vi "Main.vi"() -> ()   [LabVIEW 2023]
uses:
  States.ctl
  System Data.ctl
  <vilib>/NI/Modbus Library/API/Master/Modbus Master.lvclass
  79a3c456-e4cd-4138-946e-1f307a576655.vi
  44454701-22d1-495e-97a7-b05a01e852b1.vi
  201a4777-ac33-490a-a616-c2a30b6a5525.vi
  0b243ea3-5714-4a42-89da-e34ccc22f44d.vi
  d4d9ab7c-afa5-4cc4-8e9e-5fa7235f49d3.vi
  d383db1f-ab98-46e8-8b04-d05cf59c4aeb.vi
  <vilib>/Utility/config.llb/Read Key (String).vi
  RS485/RS485.lvlib
  <vilib>/Utility/config.llb/NI_LVConfig.lvlib
  Arduino code/Serial_communication.lvlib
panel:
  in  "Izabrana varijanta":string
  in  "Select Variant":bool=TRUE
  in  "Status":bool
  in  "Stop":bool
  out "error out":errorcluster
  in  "Test":T1(array[cluster])
  in  "Dostupne varijante":string(combo)
  in  "error in":errorcluster
  in  "START":bool
  out "Monitor":string
  # "Ime testa"
  # "Donja \ngranica"
  # "Izmerena\nvrednost"
  # "Gornja \ngranica"
  # "Rezultat\ntesta"
  # "Rezultat testiranja :"
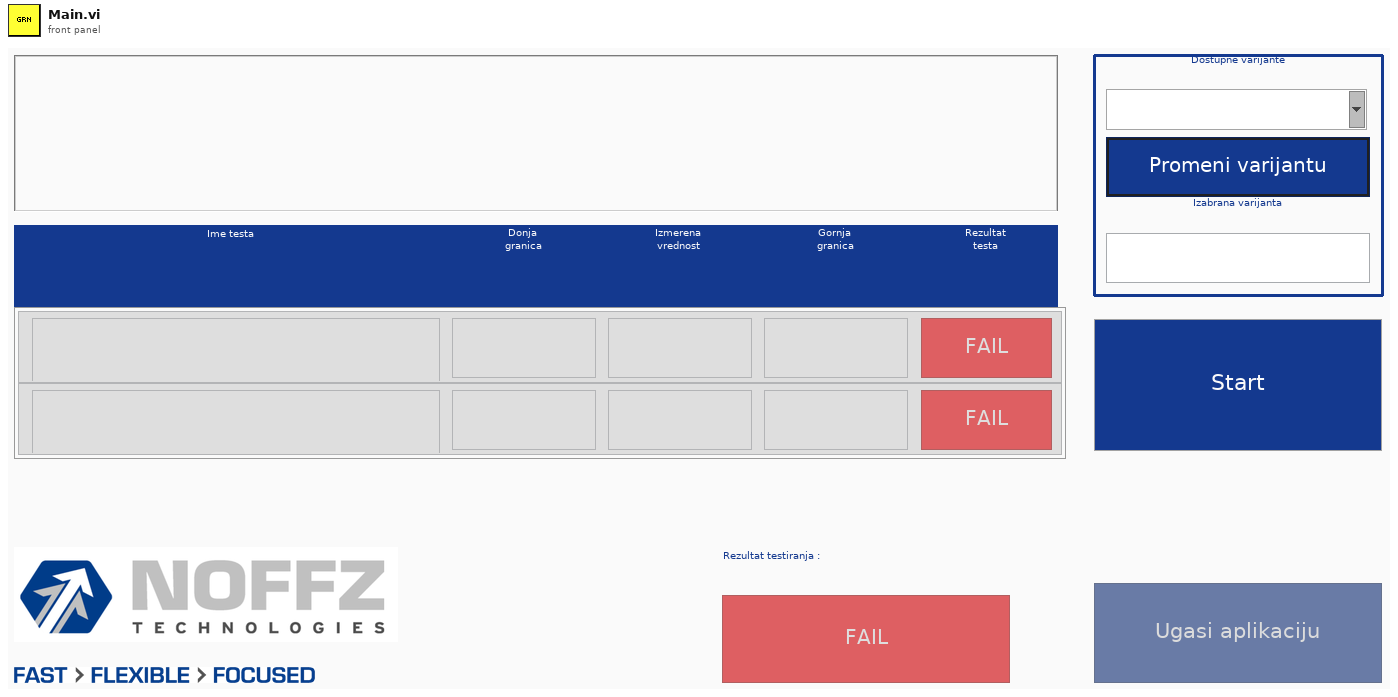
[diagram p1: front panel]
types:
  T1 = cluster{"TestName":string, "LOW":string, "MEAS":string, "HIGH":string, "Status":bool}[]
  T2 = cluster{"TestName":string, "LOW":string, "MEAS":string, "HIGH":string, "STATUS":bool}[]
  T3 = typedef "System Data.ctl" = cluster{"RS485 reference":refnum<class "Modbus Master.lvclass">, "Testing Status":bool, "Selected Variant":string, "Number Of tests":i32, "Test Names":string[], "Test Results":bool[], "Test Limits":cluster{"Low Limit":dbl, "High Limit":dbl, "GELE":bool}[], "Current test":i32, "Test Values":dbl[], "ArduinoRef":refnum<visa-resource-name>}
  T4 = typedef "States.ctl" = enum16{"Initialize", "Select Variant", "Idle", "Start Test", "Test", "Result", "Deinitialize"}
  T5 = enum8{"Enabled", "Disabled", "Disabled and Grayed Out"}
  T6 = cluster{"TestName":string, "LOW":string, "MEAS":string, "HIGH":string, "Status":bool}
  T7 = cluster{"TestName":string, "LOW":string, "MEAS":string, "HIGH":string, "STATUS":bool}
  T8 = typedef "NI_LVConfig.lvlib/Config Data RefNum.ctl" = refnum<k1>
  T9 = cluster{"Low Limit":dbl, "High Limit":dbl, "GELE":bool}[]
  T10 = cluster{"Low Limit":dbl, "High Limit":dbl, "GELE":bool}
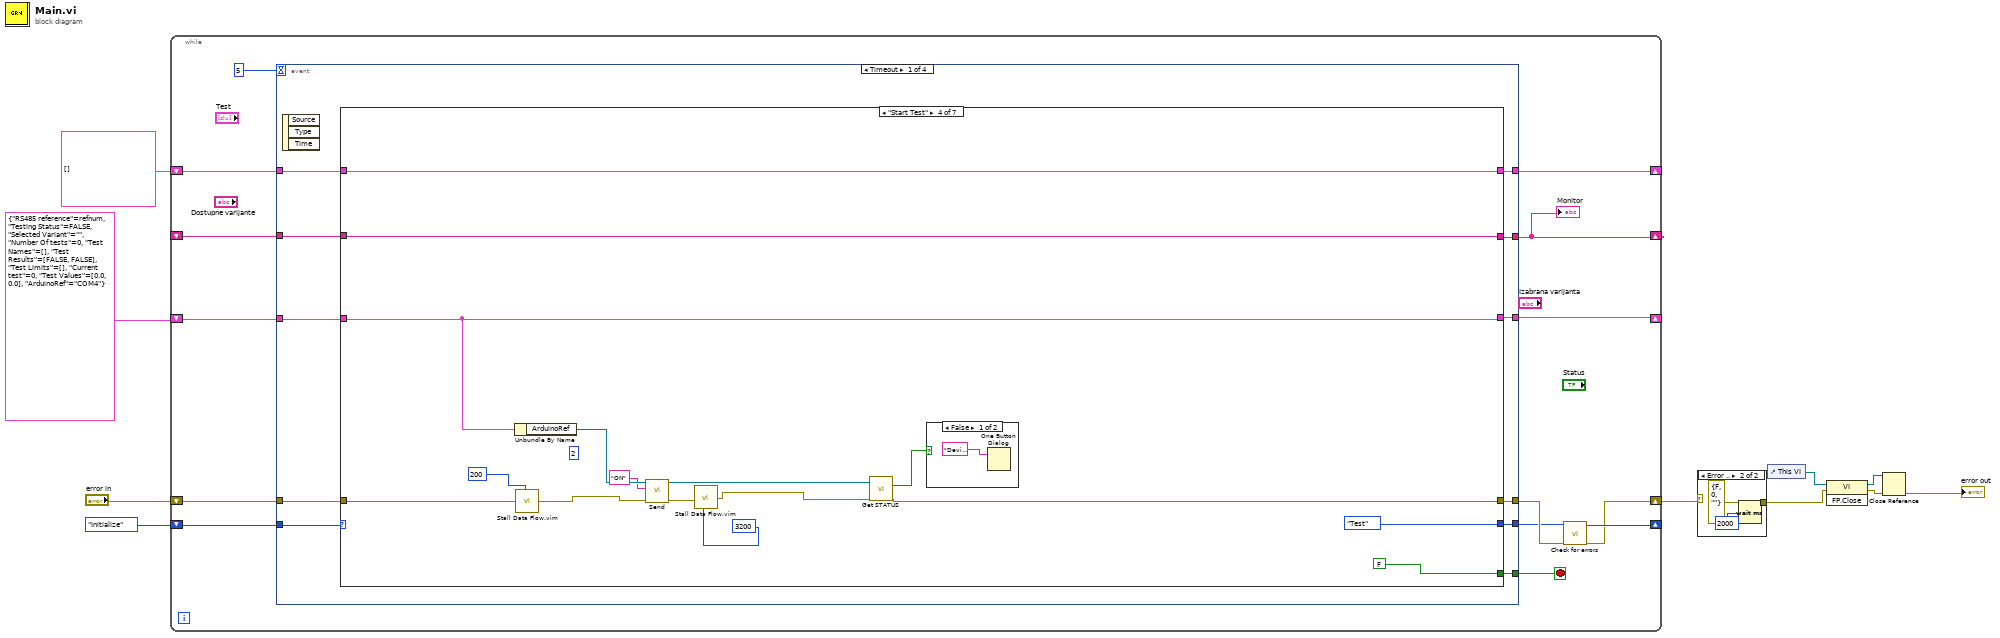
[diagram p0: block diagram]
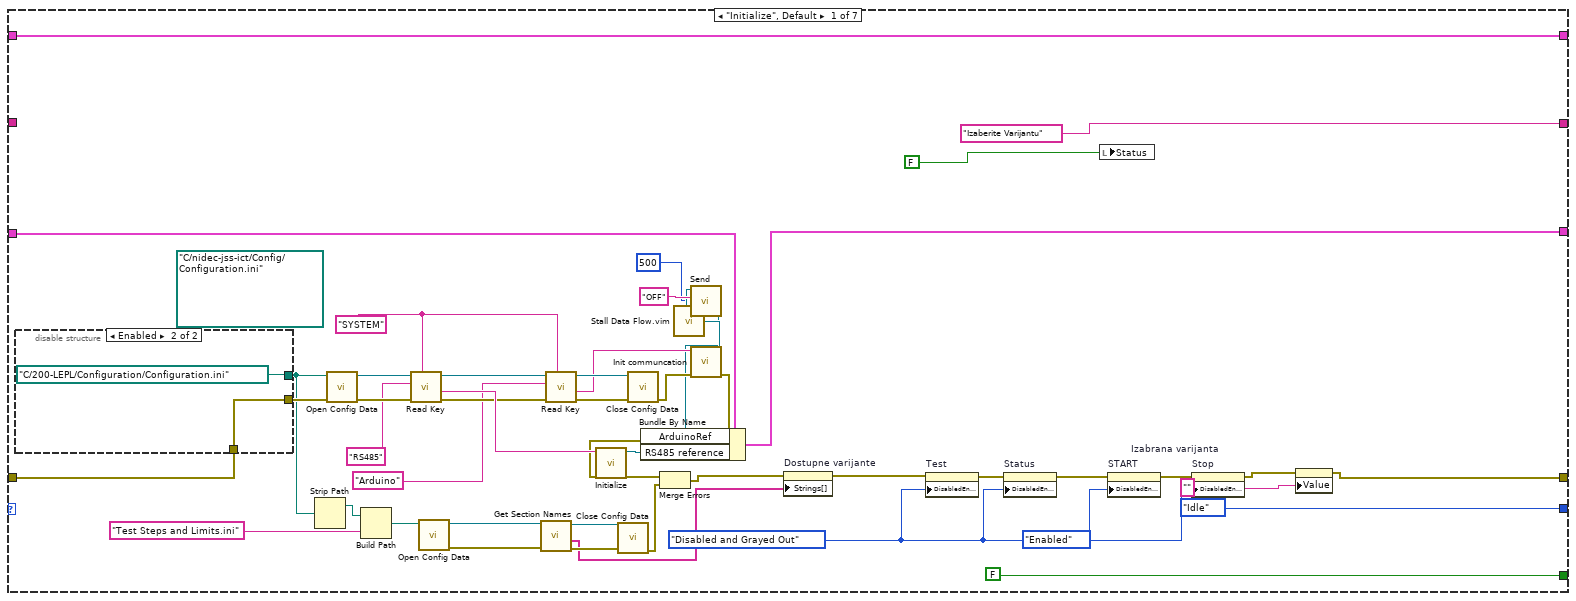
[diagram p3: hidden frame]
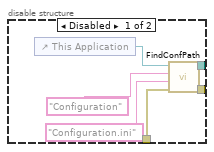
[diagram p4: hidden frame]
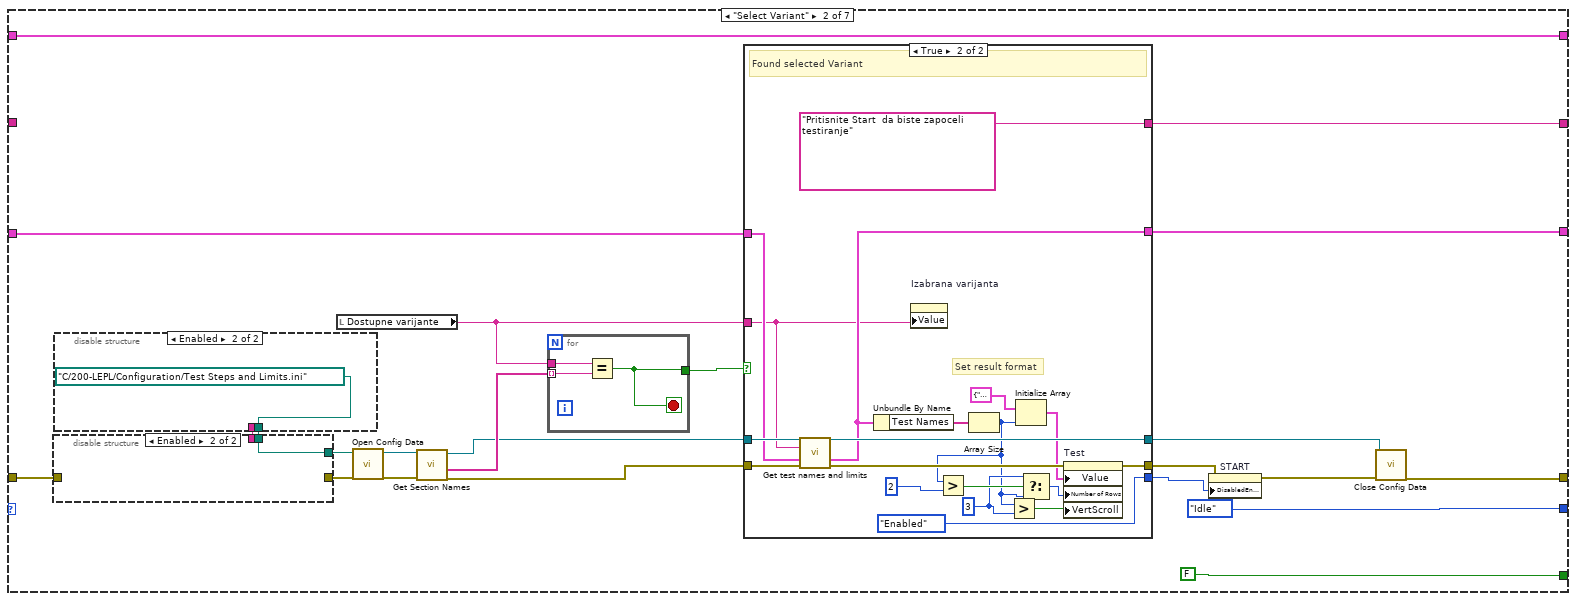
[diagram p5: hidden frame]
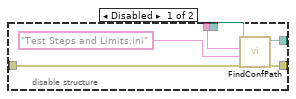
[diagram p6: hidden frame]
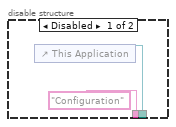
[diagram p7: hidden frame]
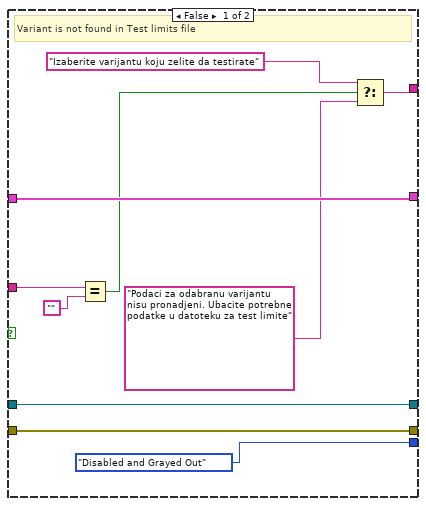
[diagram p8: hidden frame]
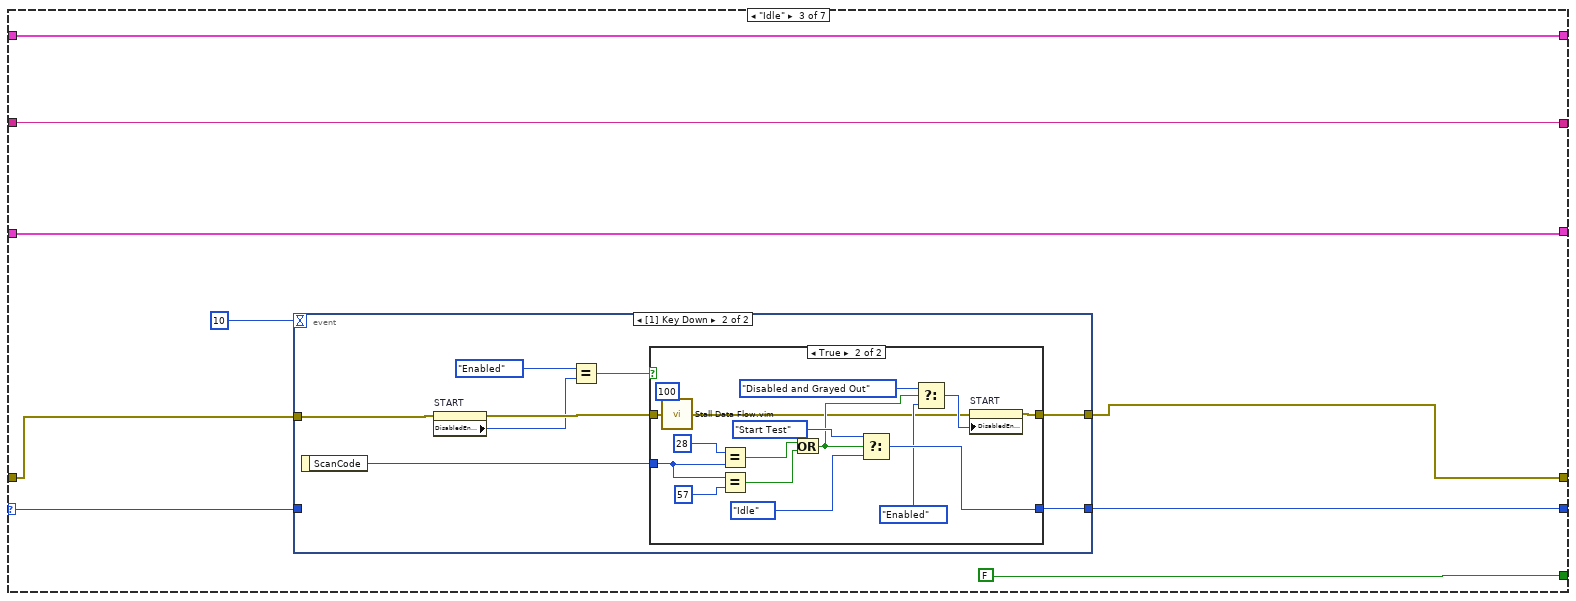
[diagram p9: hidden frame]
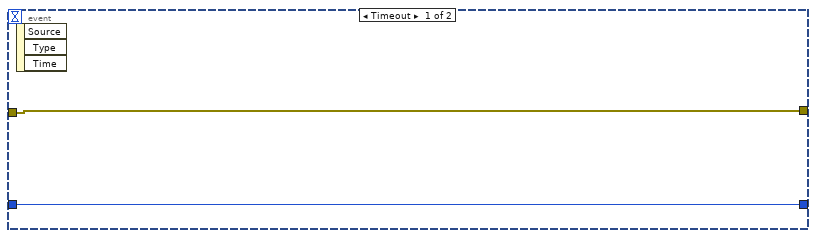
[diagram p10: hidden frame]
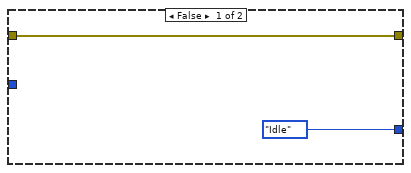
[diagram p11: hidden frame]
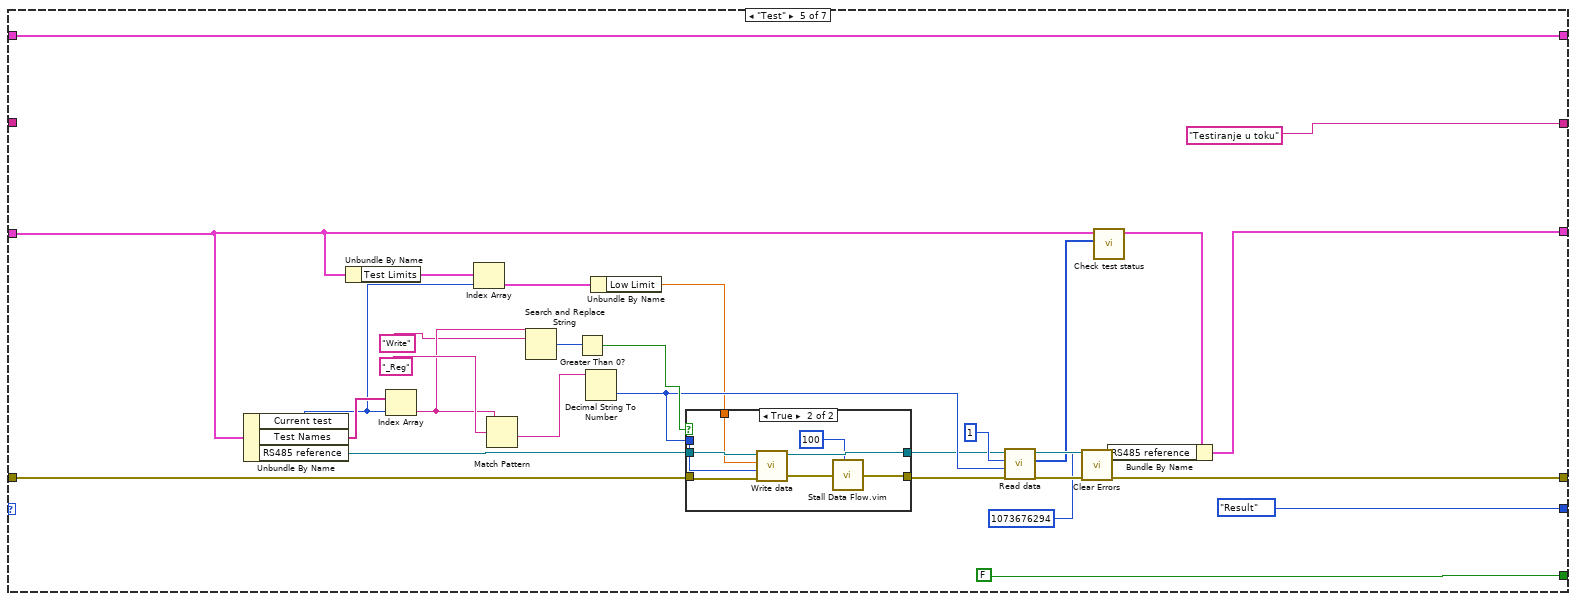
[diagram p13: hidden frame]
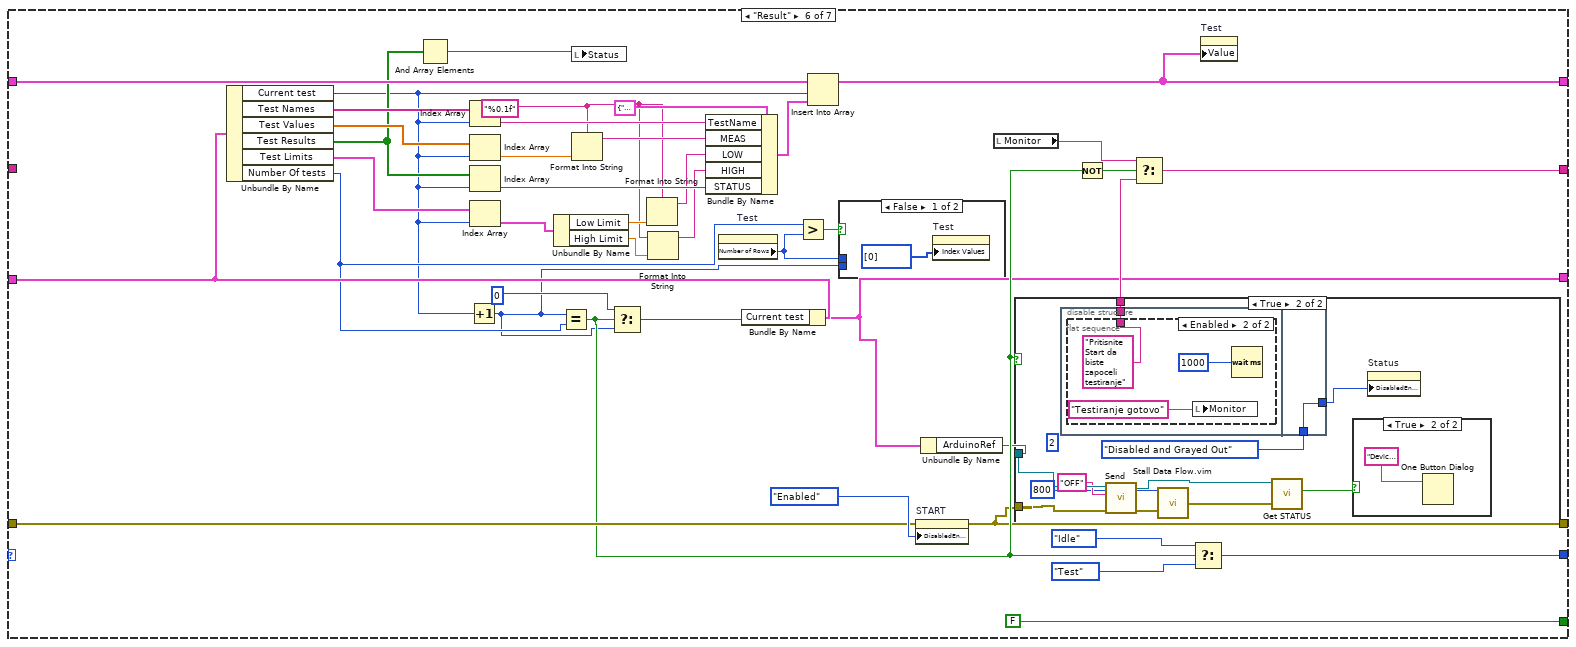
[diagram p15: hidden frame]
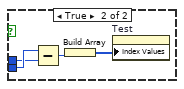
[diagram p16: hidden frame]
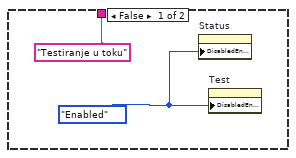
[diagram p17: hidden frame]
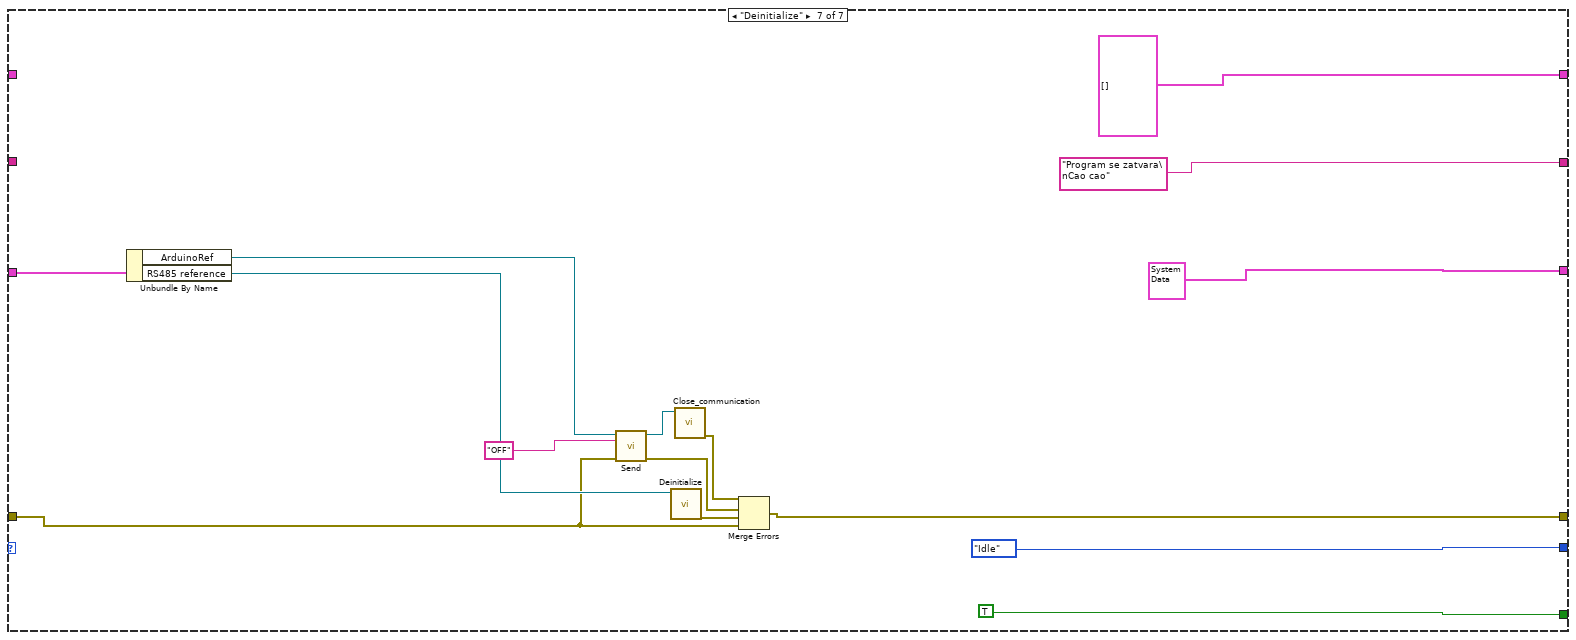
[diagram p20: hidden frame]
diagram:
  n1 = while {
    shift-right: [w12] -> w3
    shift-left: "error in" -> [w22]
    shift-right: [w20] -> _
    shift-left: T3 {"RS485 reference"=refnum, "Testing Status"=FALSE, "Selected Variant"="", "Number Of tests"=0, "Test Names"=[], "Test Results"=[FALSE, FALSE], "Test Limits"=[], "Current test"=0, "Test Values"=[0.0, 0.0], "ArduinoRef"="COM4"} -> [w21]
    shift-right: [w16] -> _
    shift-left: States."Initialize" -> [w23]
    shift-right: [w11] -> _
    shift-left: T2 [] ("Test") -> [w15]
    shift-right: [w14] -> _
    shift-left: _ -> [w13]
    stop <- w19 stop-if-true
    n2 = event shown="[0] Timeout" {
      selector: _ -> [_ _ _ _]
      dyn-events: _ -> [_ _ _ _]
      timeout: 5 -> [_ _ _ _]
      tunnel: w23 -> [w35 _ _ _]
      tunnel: w22 -> [w34 w334 w341 w347]
      tunnel: w21 -> [w33 w333 w342 w350]
      tunnel: [w32 w334 w340 w346] -> w18
      tunnel: [w31 w333 w342 w350] -> w20
      tunnel: [w30 FALSE FALSE FALSE] -> w19
      tunnel: [w29 States."Select Variant" States."Start Test" States."Deinitialize"] -> w17
      tunnel: [w28 w331 w338 w349] -> w11
      tunnel: w15 -> [w27 w331 w338 w349]
      tunnel: [w26 w332 w337 w348] -> w14
      tunnel: w13 -> [w25 w332 w337 w348]
      event Timeout {
        n3 = event-data() -> ()  [unwired: 1 in, 3 out]
        n4 = case shown="\"Start Test\"" w35 {
          selector: w35 -> [_ _ w158 _ _ _ _]
          tunnel: w34 -> [w72 w113 w161 w201 w217 w289 w318]
          tunnel: w33 -> [w79 w105 w166 w208 w222 w273 w327]
          tunnel: [w50 w103 w160 w203 w213 w253 w323] -> w32
          tunnel: [w77 w104 w166 w208 w233 w252 T3 {"RS485 reference"=refnum, "Testing Status"=FALSE, "Selected Variant"="", "Number Of tests"=0, "Test Names"=[], "Test Results"=[], "Test Limits"=[], "Current test"=0, "Test Values"=[], "ArduinoRef"="COM4"}] -> w31
          tunnel: [FALSE FALSE FALSE FALSE FALSE FALSE TRUE] -> w30
          tunnel: [States."Idle" States."Idle" w159 States."Test" States."Result" w268 States."Idle"] -> w29
          tunnel: [w58 w94 w164 w210 w238 w259 T2 [] ("Test")] -> w28
          tunnel: w27 -> [w58 w94 w164 w210 w238 w288 _]
          tunnel: ["Izaberite Varijantu" ("Monitor") w93 w163 w209 "Testiranje u toku" ("message") w266 "Program se zatvara\nCao cao" ("message")] -> w26
          tunnel: w25 -> [_ _ w163 w209 _ _ _]
          frame "Initialize", Default {
            w53 = T5."Disabled and Grayed Out" ("Disabled")
            w44 = "SYSTEM" ("key")
            (unwired) path "C:/nidec-jss-ict/Config/Configuration.ini" ("configuration file path")
            n5 = disable-structure shown="Enabled" {
              disable-tunnel: [w88 w92] -> w84
              disable-tunnel: w72 -> [w87 w92]
              disable-tunnel: [w85 path "C:/200-LEPL/Configuration/Configuration.ini" ("conf path")] -> w71
              frame Disabled {
                n6 = control-ref of="This Application"() -> (w86:refnum<vi>)
                n7 = call "FindConfPath.vi"("error in"=w87, "FileName"="Configuration.ini", "SubFolder"="Configuration", "Application in"=w86) -> ("error out"=w88:errorcluster, "conf path"=w85:path)  [unwired: 6 in]
              }
              frame Enabled {
              }
            }
            n8 = Strip Path(path=w71) -> (stripped path=w70:path)  [unwired: 1 out]
            n9 = call <vilib>:"Open Config Data.vi"("error in (no error)"=w84, "configuration file path"=w71) -> ("error out"=w82:errorcluster, "refnum"=w83:T8)  [unwired: 7 in, 1 out]
            n10 = Build Path(base path=w70, name or relative path="Test Steps and Limits.ini" ("FileName")) -> (appended path=w68:path)
            n11 = call-poly <vilib>:"Read Key.vi"("section"=w44, "error in (no error)"=w82, "key"="RS485" ("default value"), "refnum"=w83) -> ("error out"=w47:errorcluster, "value"=w80:string, "refnum out"=w49:T8)  [unwired: 4 in, 1 out]
            n12 = call <vilib>:"Open Config Data.vi"("configuration file path"=w68) -> ("error out"=w74:errorcluster, "refnum"=w73:T8)  [unwired: 8 in, 1 out]
            n13 = call <vilib>:"Get Section Names.vi"("error in (no error)"=w74, "refnum"=w73) -> ("error out"=w67:errorcluster, "section names"=w63:string[], "refnum out"=w66:T8)  [unwired: 7 in]
            n14 = call-poly <vilib>:"Read Key.vi"("section"=w44, "error in (no error)"=w47, "key"="Arduino", "refnum"=w49) -> ("error out"=w46:errorcluster, "value"=w41:string, "refnum out"=w48:T8)  [unwired: 4 in, 1 out]
            n15 = call <vilib>:"Close Config Data.vi"("error in (no error)"=w67, "refnum"=w66) -> ("error out"=w64:errorcluster)  [unwired: 8 in, 1 out]
            n16 = call <vilib>:"Close Config Data.vi"("error in (no error)"=w46, "refnum"=w48) -> ("error out"=w43:errorcluster)  [unwired: 8 in, 1 out]
            n17 = call "Init communcation.vi"("error in (no error)"=w43, "COM port"=w41) -> ("error out"=w42:errorcluster, "VISA Refnum out"=w40:refnum<visa-resource-name>)  [unwired: 8 in]
            n18 = call "Initialize.vi"("error in"=w42, "NI name"=w80) -> ("error out"=w65:errorcluster, "Modbus master out"=w78:refnum<class "Modbus Master.lvclass">)  [unwired: 8 in]
            n19 = Merge Errors(w65, w64) -> (w57:errorcluster)
            n20 = call "Stall Data Flow.vim"("value in"=w40, "milliseconds to wait"=u32 500) -> ("value out"=w37:refnum<visa-resource-name>)  [unwired: 1 out]
            n21 = call "Send.vi"("Command"="OFF", "VISA Refnum in"=w37) -> ("VISA Refnum out"=w39:refnum<visa-resource-name>)  [unwired: 8 in, 1 out]
            n22 = Bundle By Name(cluster=w79, "ArduinoRef"=w39, "RS485 reference"=w78) -> (w77:T3)
            n23 = property on="Dostupne varijante" class="CmbBox"(error in=w57, "Strings[]"=w63) -> (error out=w55:errorcluster)  [unwired: 1 in, 1 out]
            n24 = property on="Test" class="Arr (strict)"(error in=w55, "DisabledEnum"=w53) -> (error out=w56:errorcluster)  [unwired: 1 in, 1 out]
            n25 = property on="Status" class="Bool (strict)"(error in=w56, "DisabledEnum"=w53) -> (error out=w54:errorcluster)  [unwired: 1 in, 1 out]
            n26 = local write "Status"(FALSE ("REZULTAT TESTIRANJA :")) -> ()
            n27 = property on="START" class="Bool"(error in=w54, "DisabledEnum"=w53) -> (error out=w60:errorcluster)  [unwired: 1 in, 1 out]
            n28 = property on="Stop" class="Bool"(error in=w60, "DisabledEnum"=T5."Enabled" ("Disabled")) -> (error out=w51:errorcluster)  [unwired: 1 in, 1 out]
            n29 = property on="Izabrana varijanta" class="Str"(error in=w51, "Value"="" ("Izabrana varijanta")) -> (error out=w50:errorcluster)  [unwired: 1 in, 1 out]
          }
          frame "Select Variant" {
            n30 = disable-structure shown="Enabled" {
              disable-tunnel: ["Configuration" ("SubFolder") _] -> w115
              disable-tunnel: [w123 path "C:/200-LEPL/Configuration/Test Steps and Limits.ini" ("conf path")] -> w114
              frame Disabled {
                n31 = control-ref of="This Application"() -> (w123:refnum<vi>)
              }
              frame Enabled {
              }
            }
            n32 = disable-structure shown="Enabled" {
              disable-tunnel: w115 -> [w121 _]
              disable-tunnel: w114 -> [w119 w122]
              disable-tunnel: w113 -> [w118 _]
              disable-tunnel: [w117 w122] -> w112
              disable-tunnel: [w116 _] -> w111
              frame Disabled {
                n33 = call "FindConfPath.vi"("error in"=w118, "FileName"="Test Steps and Limits.ini", "SubFolder"=w121, "Application in"=w119) -> ("error out"=w116:errorcluster, "conf path"=w117:path)  [unwired: 6 in]
              }
              frame Enabled {
              }
            }
            n34 = local read "Dostupne varijante"() -> (w106:string)
            n35 = call <vilib>:"Open Config Data.vi"("error in (no error)"=w111, "configuration file path"=w112) -> ("error out"=w110:errorcluster, "refnum"=w109:T8)  [unwired: 7 in, 1 out]
            n36 = call <vilib>:"Get Section Names.vi"("error in (no error)"=w110, "refnum"=w109) -> ("error out"=w95:errorcluster, "section names"=w108:string[], "refnum out"=w107:T8)  [unwired: 7 in]
            n37 = for {
              tunnel: w108 -> [w157] mode=indexing
              tunnel: w106 -> [w156]
              tunnel: [w155] -> w99
              stop <- w155 stop-if-true
              n38 = Equal?(x=w156, y=w157) -> (x = y?=w155:bool)
            }
            n39 = case shown="True" w99 {
              tunnel: w107 -> [w135 w154]
              tunnel: w106 -> [w131 w136]
              tunnel: w105 -> [w134 w150]
              tunnel: [w134 w148] -> w104
              tunnel: [w132 w146] -> w98
              tunnel: [w135 w153] -> w102
              tunnel: [T5."Disabled and Grayed Out" ("Disabled") T5."Enabled" ("Disabled")] -> w96
              tunnel: w95 -> [w132 w151]
              tunnel: [w127 "Pritisnite Start  da biste zapoceli testiranje" ("message")] -> w93
              frame False {
                # "Variant is not found in Test limits file"
                n40 = Equal?(x=w131, y="") -> (x = y?=w129:bool)
                n41 = Select(t="Izaberite varijantu koju zelite da testirate", s=w129, f="Podaci za odabranu varijantu nisu pronadjeni. Ubacite potrebne podatke u datoteku za test limite" ("message")) -> (s? t:f=w127:string)
              }
              frame True {
                w139 = 3 ("y")
                # "Set result format"
                # "Found selected Variant"
                n42 = call "Get test names and limits.vi"("Refnum in"=w154, "Variant"=w136, "System data in"=w150, "error in"=w151) -> ("Refnum out"=w153:T8, "System data out"=w148:T3, "error out"=w147:errorcluster)  [unwired: 9 in]
                n43 = Unbundle By Name(w148) -> ("Test Names"=w145:string[])
                n44 = property on="Izabrana varijanta" class="Str"("Value"=w136) -> ()  [unwired: 2 in, 2 out]
                n45 = Array Size(array=w145) -> (size(s)=w138:i32)
                n46 = Greater?(x=w138, y=2) -> (0:w140:bool)
                n47 = Greater?(x=w138, y=w139) -> (0:w142:bool)
                n48 = Initialize Array(T6 {"TestName"="", "LOW"="", "MEAS"="", "HIGH"="", "Status"=FALSE} ("Test"), w138) -> (w143:T1)
                n49 = Select(t=w139, s=w140, f=w138) -> (s? t:f=w137:i32)
                n50 = property on="Test" class="Arr (strict)"(error in=w147, "Value"=w143, "Number of Rows"=w137, "VertScroll"=w142) -> (error out=w146:errorcluster)  [unwired: 1 in, 1 out]
              }
            }
            n51 = property on="START" class="Bool"(error in=w98, "DisabledEnum"=w96) -> (error out=w97:errorcluster)  [unwired: 1 in, 1 out]
            n52 = call <vilib>:"Close Config Data.vi"("error in (no error)"=w97, "refnum"=w102) -> ("error out"=w103:errorcluster)  [unwired: 8 in, 1 out]
          }
          frame "Idle" {
            n53 = event shown="[1] Key Down" {
              selector: _ -> [_ _]
              dyn-events: _ -> [_ _]
              timeout: 10 -> [_ _]
              tunnel: w161 -> [w167 w169]
              tunnel: [w167 w173] -> w160
              tunnel: [w168 w172] -> w159
              tunnel: w158 -> [w168 _]
              event Timeout {
                n54 = event-data() -> ()  [unwired: 1 in, 3 out]
              }
              event Key Down {
                n55 = event-data() -> ("ScanCode"=w174:i16)  [unwired: 1 in]
                n56 = property on="START" class="Bool"(error in=w169) -> (error out=w171:errorcluster, "DisabledEnum"=w170:T5)  [unwired: 1 in, 1 out]
                n57 = Equal?(x=T5."Enabled", y=w170) -> (x = y?=w175:bool)
                n58 = case shown="True" w175 {
                  tunnel: w174 -> [_ w189]
                  tunnel: [States."Idle" w190] -> w172
                  tunnel: w171 -> [w177 w186]
                  tunnel: [w177 w185] -> w173
                  frame False {
                  }
                  frame True {
                    n59 = call "Stall Data Flow.vim"("value in"=w186, "milliseconds to wait"=u32 100) -> ("value out"=w180:errorcluster)  [unwired: 1 out]
                    n60 = Equal?(x=i16 28, y=w189) -> (x = y?=w192:bool)
                    n61 = Equal?(x=w189, y=i16 57 ("x")) -> (x = y?=w191:bool)
                    n62 = Or(x=w192, y=w191) -> (x .or. y?=w183:bool)
                    n63 = Select(t=States."Start Test", s=w183, f=States."Idle") -> (s? t:f=w190:T4)
                    n64 = Select(t=T5."Disabled and Grayed Out" ("Disabled"), s=w183, f=T5."Enabled" ("Disabled")) -> (s? t:f=w181:T5)
                    n65 = property on="START" class="Bool"(error in=w180, "DisabledEnum"=w181) -> (error out=w185:errorcluster)  [unwired: 1 in, 1 out]
                  }
                }
              }
            }
          }
          frame "Start Test" {
            (unwired) 2
            n66 = Unbundle By Name(w208) -> ("ArduinoRef"=w205:refnum<visa-resource-name>)
            n67 = call "Stall Data Flow.vim"("value in"=w201, "milliseconds to wait"=u32 200) -> ("value out"=w197:errorcluster)  [unwired: 1 out]
            n68 = call "Send.vi"("error in (no error)"=w197, "Command"="ON", "VISA Refnum in"=w205) -> ("error out"=w195:errorcluster, "VISA Refnum out"=w204:refnum<visa-resource-name>)  [unwired: 7 in]
            n69 = call "Stall Data Flow.vim"("value in"=w195, "milliseconds to wait"=u32 3200) -> ("value out"=w198:errorcluster)  [unwired: 1 out]
            n70 = call "Get STATUS.vi"("error in (no error)"=w198, "VISA Refnum in"=w204) -> ("error out"=w203:errorcluster, "LED ON"=w202:bool)  [unwired: 6 in, 2 out]
            n71 = case shown="False" w202 {
              frame False {
                n72 = One Button Dialog(message="Device did not turn ON. Please close the program and open it again") -> ()  [unwired: 1 in, 1 out]
              }
              frame True {
              }
            }
          }
          frame "Test" {
            n73 = Unbundle By Name(w222) -> ("Current test"=w220:i32, "Test Names"=w237:string[], "RS485 reference"=w224:refnum<class "Modbus Master.lvclass">)
            n74 = Unbundle By Name(w222) -> ("Test Limits"=w221:T9)
            n75 = Index Array(array=w237, index=w220) -> (element=w228:string)
            n76 = Index Array(array=w221, index=w220) -> (element=w219:T10)
            n77 = Match Pattern(string=w228, regular expression="_Reg") -> (after substring=w235:string)  [unwired: 1 in, 3 out]
            n78 = Search and Replace String(input string=w228, search string="Write") -> (number of replacements=w226:i32)  [unwired: 6 in, 3 out]
            n79 = Greater Than 0?(x=w226) -> (x > 0?=w225:bool)
            n80 = Decimal String To Number(string=w235) -> (number=w223:i32)  [unwired: 2 in, 1 out]
            n81 = Unbundle By Name(w219) -> ("Low Limit"=w218:dbl)
            n82 = case shown="True" w225 {
              tunnel: w224 -> [w242 w250]
              tunnel: [w242 w249] -> w215
              tunnel: w223 -> [_ w248]
              tunnel: w218 -> [_ w247]
              tunnel: w217 -> [w241 w246]
              tunnel: [w241 w244] -> w214
              frame False {
              }
              frame True {
                n83 = call "Write data.vi"("error in"=w246, "starting address"=w248, "register value to write"=w247, "Modbus master in"=w250) -> ("error out"=w245:errorcluster, "Modbus master out"=w249:refnum<class "Modbus Master.lvclass">)  [unwired: 6 in]
                n84 = call "Stall Data Flow.vim"("value in"=w245, "milliseconds to wait"=u32 100) -> ("value out"=w244:errorcluster)  [unwired: 1 out]
              }
            }
            n85 = call "Read data.vi"("error in"=w214, "starting address"=w223, "number of inputs"=u16 1, "Modbus master in"=w215) -> ("error out"=w234:errorcluster, "register values"=w230:u16[], "Modbus master out"=w232:refnum<class "Modbus Master.lvclass">)  [unwired: 5 in]
            n86 = call <vilib>:"Clear Errors.vi"("error in (no error)"=w234, "specific error code to clear (0: all)"=1073676294) -> ("error out"=w213:errorcluster)  [unwired: 4 in, 1 out]
            n87 = call "Check test status.vi"("register values"=w230, "System data in"=w222) -> ("System data out"=w231:T3)  [unwired: 9 in]
            n88 = Bundle By Name(cluster=w231, "RS485 reference"=w232) -> (w233:T3)
          }
          frame "Result" {
            w263 = "%0.1f" ("format string")
            n89 = Unbundle By Name(w273) -> ("Current test"=w256:i32, "Test Names"=w286:string[], "Test Values"=w284:dbl[], "Test Results"=w264:bool[], "Test Limits"=w280:T9, "Number Of tests"=w258:i32)
            n90 = And Array Elements(Boolean array=w264) -> (logical AND=w265:bool)
            n91 = Increment(x=w256) -> (x+1=w255:i32)
            n92 = Index Array(array=w286, index=w256) -> (element=w285:string)
            n93 = Index Array(array=w284, index=w256) -> (element=w283:dbl)
            n94 = Index Array(array=w264, index=w256) -> (element=w281:bool)
            n95 = Index Array(array=w280, index=w256) -> (element=w279:T10)
            n96 = Unbundle By Name(w279) -> ("Low Limit"=w278:dbl, "High Limit"=w277:dbl)
            n97 = Equal?(x=w255, y=w258) -> (x = y?=w261:bool)
            n98 = local write "Status"(w265) -> ()
            n99 = Format Into String(format string=w263, w283) -> (resulting string=w282:string)  [unwired: 2 in, 1 out]
            n100 = Select(t=0, s=w261, f=w255) -> (s? t:f=w271:i32)
            n101 = Format Into String(format string=w263, w278) -> (resulting string=w276:string)  [unwired: 2 in, 1 out]
            n102 = Format Into String(format string=w263, w277) -> (resulting string=w275:string)  [unwired: 2 in, 1 out]
            n103 = Bundle By Name(cluster=T7 {"TestName"="", "LOW"="", "MEAS"="", "HIGH"="", "STATUS"=FALSE} ("new element/subarray"), "TestName"=w285, "MEAS"=w282, "LOW"=w276, "HIGH"=w275, "STATUS"=w281) -> (w274:T7)
            n104 = property on="Test" class="Arr (strict)"() -> ("Number of Rows"=w254:u32)  [unwired: 2 in, 2 out]
            n105 = Bundle By Name(cluster=w273, "Current test"=w271) -> (w252:T3)
            n106 = Greater?(x=w258, y=w254) -> (0:w257:bool)
            n107 = Insert Into Array(array=w288, index=w256, new element=w274) -> (w259:T2)
            n108 = case shown="False" w257 {
              tunnel: w255 -> [_ w296]
              tunnel: w254 -> [_ w295]
              frame False {
                n109 = property on="Test" class="Arr (strict)"("Index Values"=u32[] [0]) -> ()  [unwired: 2 in, 2 out]
              }
              frame True {
                n110 = Subtract(x=w296, y=w295) -> (x-y=w294:u32)
                n111 = Build Array(w294) -> (w293:u32[])
                n112 = property on="Test" class="Arr (strict)"("Index Values"=w293) -> ()  [unwired: 2 in, 2 out]
              }
            }
            n113 = property on="START" class="Bool"(error in=w289, "DisabledEnum"=T5."Enabled" ("Disabled")) -> (error out=w253:errorcluster)  [unwired: 1 in, 1 out]
            n114 = Unbundle By Name(w252) -> ("ArduinoRef"=w251:refnum<visa-resource-name>)
            n115 = local read "Monitor"() -> (w267:string)
            n116 = case shown="True" w261 {
              tunnel: ["Testiranje u toku" ("message") w309] -> w260
              tunnel: w253 -> [_ w302]
              tunnel: w251 -> [_ w306]
              frame False {
                w298 = T5."Enabled" ("Disabled")
                n117 = property on="Status" class="Bool (strict)"("DisabledEnum"=w298) -> ()  [unwired: 2 in, 2 out]
                n118 = property on="Test" class="Arr (strict)"("DisabledEnum"=w298) -> ()  [unwired: 2 in, 2 out]
              }
              frame True {
                (unwired) 2
                n119 = flat-sequence {
                  tunnel: [w311] -> w309
                  tunnel: [w315] -> w307
                  tunnel: T5."Disabled and Grayed Out" ("Disabled") -> [w315]
                  frame #0 {
                    n120 = disable-structure shown="Enabled" {
                      disable-tunnel: [_ "Pritisnite Start da biste zapoceli testiranje" ("message")] -> w311
                      frame Disabled {
                      }
                      frame Enabled {
                        n121 = local write "Monitor"("Testiranje gotovo" ("Monitor")) -> ()
                        n122 = Wait (ms)(milliseconds to wait=u32 1000) -> ()  [unwired: 1 out]
                      }
                    }
                  }
                  frame #1 {
                  }
                }
                n123 = call "Send.vi"("error in (no error)"=w302, "Command"="OFF", "VISA Refnum in"=w306) -> ("error out"=w300:errorcluster, "VISA Refnum out"=w305:refnum<visa-resource-name>)  [unwired: 7 in]
                n124 = call "Stall Data Flow.vim"("value in"=w300, "milliseconds to wait"=u32 800) -> ("value out"=w303:errorcluster)  [unwired: 1 out]
                n125 = call "Get STATUS.vi"("error in (no error)"=w303, "VISA Refnum in"=w305) -> ("LED ON"=w304:bool)  [unwired: 6 in, 3 out]
                n126 = case shown="True" w304 {
                  frame False {
                  }
                  frame True {
                    n127 = One Button Dialog(message="Device did not reset\nPlease close the prorgam and open it again") -> ()  [unwired: 1 in, 1 out]
                  }
                }
                n128 = property on="Status" class="Bool (strict)"("DisabledEnum"=w307) -> ()  [unwired: 2 in, 2 out]
              }
            }
            n129 = Not(x=w261) -> (.not. x?=w262:bool)
            n130 = Select(t=w267, s=w262, f=w260) -> (s? t:f=w266:string)
            n131 = Select(t=States."Idle", s=w261, f=States."Test") -> (s? t:f=w268:T4)
            n132 = property on="Test" class="Arr (strict)"("Value"=w259) -> ()  [unwired: 2 in, 2 out]
          }
          frame "Deinitialize" {
            n133 = Unbundle By Name(w327) -> ("ArduinoRef"=w321:refnum<visa-resource-name>, "RS485 reference"=w330:refnum<class "Modbus Master.lvclass">)
            n134 = call "Send.vi"("error in (no error)"=w318, "Command"="OFF", "VISA Refnum in"=w321) -> ("error out"=w316:errorcluster, "VISA Refnum out"=w320:refnum<visa-resource-name>)  [unwired: 7 in]
            n135 = call "Deinitialize.vi"("Modbus master in"=w330) -> ("error out"=w324:errorcluster)  [unwired: 10 in]
            n136 = call "Close_communication.vi"("VISA Refnum in"=w320) -> ("error out"=w317:errorcluster)  [unwired: 10 in]
            n137 = Merge Errors(w317, w316, w324, w318) -> (w323:errorcluster)
          }
        }
      }
      event "Select Variant": Value Change {
        n138 = event-data() -> ()  [unwired: 1 in, 6 out]
      }
      event "START": Value Change {
        n139 = event-data() -> ()  [unwired: 1 in, 2 out]
        n140 = property on="START" class="Bool"(error in=w341, "DisabledEnum"=T5."Disabled and Grayed Out" ("Disabled")) -> (error out=w340:errorcluster)  [unwired: 1 in, 1 out]
      }
      event "Stop": Value Change {
        n141 = event-data() -> ()  [unwired: 1 in, 6 out]
        n142 = property on="Stop" class="Bool"(error in=w347, "DisabledEnum"=T5."Disabled and Grayed Out" ("Disabled")) -> (error out=w346:errorcluster)  [unwired: 1 in, 1 out]
      }
    }
    "Monitor" <- w14
    n143 = call "Check for errors.vi"("error in"=w18, "Next state in"=w17) -> ("error out"=w12:errorcluster, "Next state out"=w16:T4)  [unwired: 8 in]
  }
  n144 = case shown="Error .." w3 {
    selector: w3 -> [w353 _]
    tunnel: [w353 errorcluster {"status"=FALSE, "code"=0, "source"=""} ("error in (no error)")] -> w1
    frame No Error {
    }
    frame Error {
      n145 = Wait (ms)(milliseconds to wait=u32 2000) -> ()  [unwired: 1 out]
    }
  }
  n146 = control-ref of="This VI"() -> (w6:refnum<vi>)
  n147 = invoke class="VI" method="FP.Close"(reference=w6, error in=w1) -> (reference out=w4:refnum<vi>, error out=w5:errorcluster)  [unwired: 1 in, 1 out]
  n148 = Close Reference(reference=w4, error in (no error)=w5) -> (error out=→"error out":errorcluster)
